vi "Memory.Pointer.Bool.Read.vi"(8 "error in (no error)":errorcluster, 10 "value":bool, 11 "U64 Pointer in":refnum<class "Memory.Pointer.Bool.lvclass">) -> (0 "error out":errorcluster, 2 "value out":bool, 3 "U64 Pointer out":refnum<class "Memory.Pointer.Bool.lvclass">)   [LabVIEW 2016, in "LabVIEW Memory Manager.lvlib" / "Memory.Pointer.Bool.lvclass"]
uses:
  Memory.Pointer.Bool.lvclass
  C:/Users/Ryan/Documents/Git/Sourcetree/LabVIEW-Memory-Manager/Source/Library/Classes/Pointer/Memory.Pointer.Void.lvclass
  Pointer/Memory.Pointer.Void.lvclass/Memory.Pointer.Void.ctl
  Pointer/Memory.Pointer.Void.lvclass
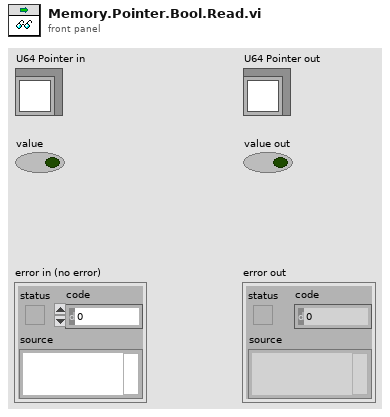
[diagram p1: front panel]
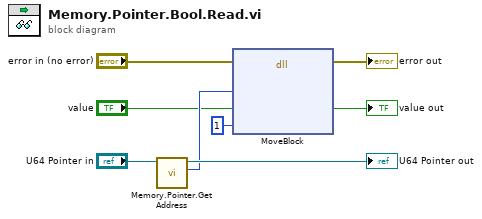
[diagram p0: block diagram]
diagram:
  n1 = call "Memory.Pointer.Get Address.vi"("Pointer in"="U64 Pointer in") -> ("address"=w2:u64, "Pointer out"=→"U64 Pointer out":refnum<class "Memory.Pointer.Bool.lvclass">)  [unwired: 8 in, 1 out]
  n2 = dll-call lib="LabVIEW" fn="MoveBlock"(error in="error in (no error)", "src"=w2, "dst"="value", "size"=u64 1) -> (error out=→"error out":errorcluster, "dst"=→"value out":bool)  [unwired: 5 in, 1 out]
